vi "WS1050_AD7747_Control_Cap_bank_Measure Ver1.0.vi"(0 "Select Com Port":refnum<visa-resource-name>="COM1", 1 "S_Value C1":dbl, 2 "S_Value C2":dbl, 3 "S_Value C3":dbl, 4 "Push Button to write Offset":bool, 7 "errorin":errorcluster, 8 "Click down to quit":bool, 9 "Push Button to Measue Cap":bool=TRUE, 12 "Mode":bool=TRUE, 14 "Push Button to Initialize AD7747":bool, 15 "CApDac_values":string[](array[string])=["900b99", "900b99", "900b9b"], 16 "Push Button to Calibrate":bool) -> (17 "Com Port Out":refnum<visa-resource-name>="COM1", 20 "C2(pF)":dbl, 21 "C1_Mesa(pF)":dbl, 22 "C2_Mesa(pF)":dbl, 23 "C3_Mesa(pF)":dbl, 24 "C1(pF)":dbl, 25 "C3(pF)":dbl, 27 "error out":errorcluster)   [LabVIEW 2017]
panel:
  # "AD7747 Control Ver1.0"
  # "Interface PIC I2C Control"
  # "Bank Cap Measurements"
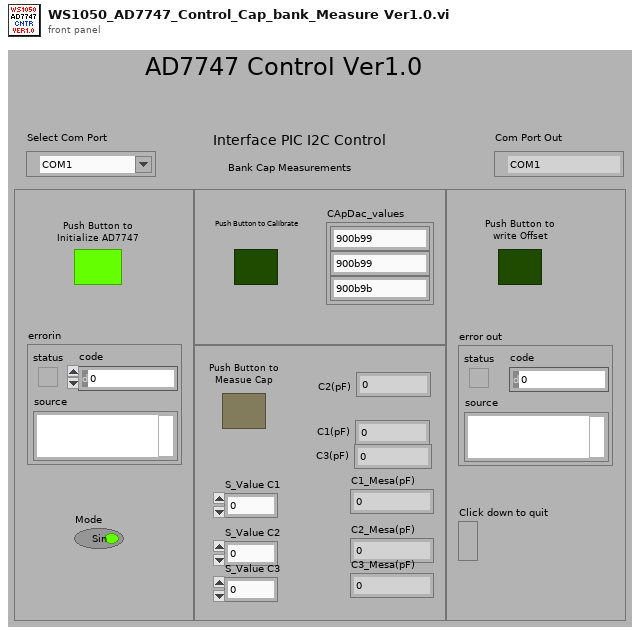
[diagram p1: front panel]
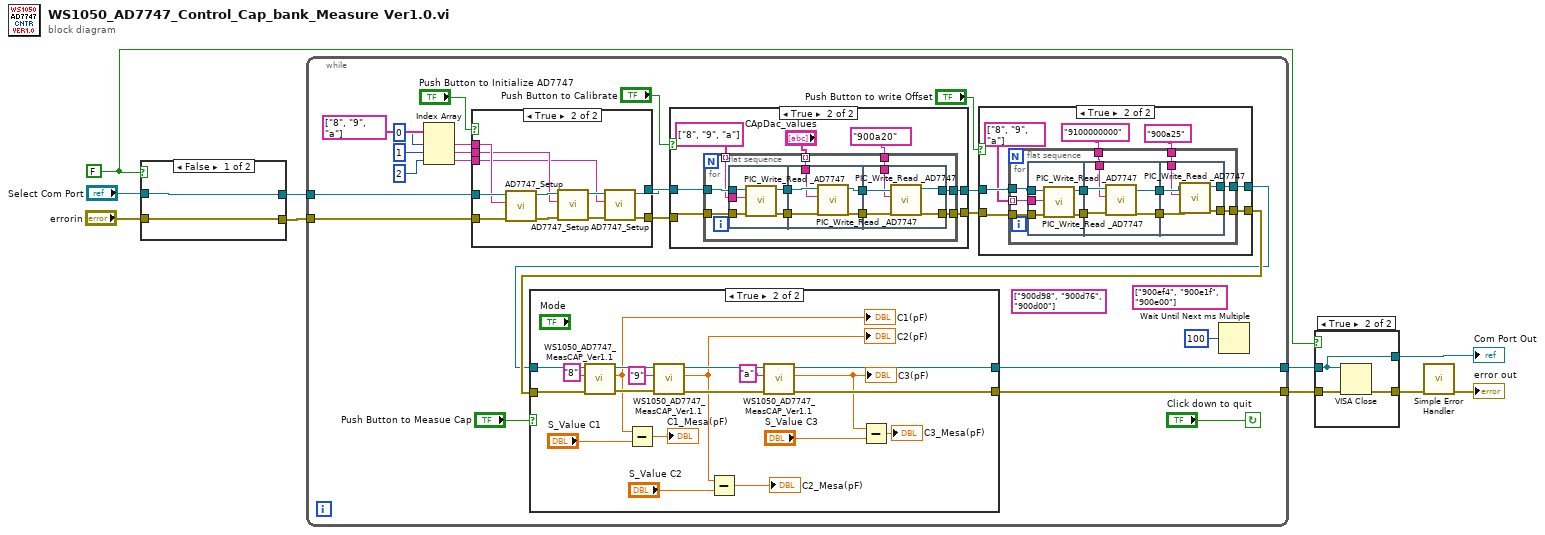
[diagram p0: block diagram]
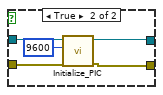
[diagram p3: hidden frame]
diagram:
  w5 = FALSE
  n1 = case shown="False" w5 {
    tunnel: [w11 w17] -> w10
    tunnel: [w12 w16] -> w9
    tunnel: "Select Com Port" -> [w12 w15]
    tunnel: "errorin" -> [w11 w13]
    frame False {
    }
    frame True {
      n2 = call "Initialize_PIC.vi"("error in (no error)"=w13, "baud rate"=u32 9600, "Select Com Port"=w15) -> ("error out"=w17:errorcluster, "VISA resource name out"=w16:refnum<visa-resource-name>)  [unwired: 7 in]
    }
  }
  n3 = while {
    tunnel: w10 -> [w35]
    tunnel: w9 -> [w33]
    tunnel: [w22] -> w8
    tunnel: [w40] -> w7
    stop <- "Click down to quit" continue-if-true
    (unwired) string[] ["900ef4", "900e1f", "900e00"]
    (unwired) string[] ["900d98", "900d76", "900d00"]
    n4 = Index Array(array=string[] ["8", "9", "a"], index #1=0 ("index"), index #2=1 ("index"), index #3=2 ("index")) -> (element #1=w36:string, element #2=w29:string, element #3=w28:string)
    n5 = case shown="True" "Push Button to Initialize AD7747" {
      tunnel: w35 -> [w111 w122]
      tunnel: [w111 w112] -> w23
      tunnel: w33 -> [w110 w121]
      tunnel: w36 -> [_ w116]
      tunnel: w29 -> [_ w115]
      tunnel: w28 -> [_ w114]
      tunnel: [w110 w113] -> w20
      frame False {
      }
      frame True {
        n6 = call "AD7747_Setup.vi"("error in"=w122, "AD7747_Number"=w116, "Control"=w121) -> ("error out"=w120:errorcluster, "Control out"=w119:refnum<visa-resource-name>)  [unwired: 6 in, 1 out]
        n7 = call "AD7747_Setup.vi"("error in"=w120, "AD7747_Number"=w115, "Control"=w119) -> ("error out"=w118:errorcluster, "Control out"=w117:refnum<visa-resource-name>)  [unwired: 6 in, 1 out]
        n8 = call "AD7747_Setup.vi"("error in"=w118, "AD7747_Number"=w114, "Control"=w117) -> ("error out"=w112:errorcluster, "Control out"=w113:refnum<visa-resource-name>)  [unwired: 6 in, 1 out]
      }
    }
    n9 = case shown="True" "Push Button to Calibrate" {
      tunnel: [w76 w84] -> w34
      tunnel: w23 -> [w76 w81]
      tunnel: w20 -> [w77 w80]
      tunnel: [w77 w79] -> w19
      frame False {
      }
      frame True {
        n10 = for {
          tunnel: [w90] -> w84
          tunnel: w80 -> [w94]
          tunnel: w81 -> [w95]
          tunnel: string[] ["8", "9", "a"] -> [w93] mode=indexing
          tunnel: "CApDac_values" -> [w89] mode=indexing
          tunnel: [w88] -> w79
          tunnel: "900a20" ("Data_In 2") -> [w85]
          n11 = flat-sequence {
            tunnel: w95 -> [w100]
            tunnel: w94 -> [w98]
            tunnel: w93 -> [w96]
            tunnel: [w99] -> w92
            tunnel: [w97] -> w91
            tunnel: w92 -> [w104]
            tunnel: w91 -> [w105]
            tunnel: w89 -> [w102]
            tunnel: [w103] -> w87
            tunnel: [w101] -> w86
            tunnel: [w107] -> w88
            tunnel: [w109] -> w90
            tunnel: w87 -> [w109]
            tunnel: w86 -> [w108]
            tunnel: w85 -> [w106]
            frame #0 {
              n12 = call "PIC_Write_Read _AD7747.vi"("error in (no error)"=w100, "command"=w96, "Control"=w98) -> ("error out"=w99:errorcluster, "Control out"=w97:refnum<visa-resource-name>)  [unwired: 6 in, 1 out]
            }
            frame #1 {
              n13 = call "PIC_Write_Read _AD7747.vi"("error in (no error)"=w104, "command"=w102, "Control"=w105) -> ("error out"=w103:errorcluster, "Control out"=w101:refnum<visa-resource-name>)  [unwired: 6 in, 1 out]
            }
            frame #2 {
              n14 = call "PIC_Write_Read _AD7747.vi"("command"=w106, "Control"=w108) -> ("Control out"=w107:refnum<visa-resource-name>)  [unwired: 7 in, 2 out]
            }
          }
        }
      }
    }
    n15 = case shown="True" "Push Button to write Offset" {
      tunnel: w19 -> [w41 w48]
      tunnel: w34 -> [w42 w49]
      tunnel: [w42 w46] -> w21
      tunnel: [w41 w45] -> w18
      frame False {
      }
      frame True {
        n16 = for {
          tunnel: w49 -> [w50]
          tunnel: [w54] -> w46
          tunnel: w48 -> [w60]
          tunnel: string[] ["8", "9", "a"] -> [w59] mode=indexing
          tunnel: "9100000000" ("Data_In 2") -> [w53]
          tunnel: "900a25" ("Data_In 2") -> [w52]
          tunnel: [w51] -> w45
          n17 = flat-sequence {
            tunnel: w60 -> [w63]
            tunnel: w59 -> [w62]
            tunnel: [w65] -> w58
            tunnel: [w64] -> w57
            tunnel: w50 -> [w61]
            tunnel: w58 -> [w68]
            tunnel: w57 -> [w70]
            tunnel: [w67] -> w56
            tunnel: [w69] -> w55
            tunnel: w53 -> [w66]
            tunnel: w56 -> [w74]
            tunnel: w55 -> [w75]
            tunnel: [w73] -> w54
            tunnel: w52 -> [w72]
            tunnel: [w71] -> w51
            frame #0 {
              n18 = call "PIC_Write_Read _AD7747.vi"("error in (no error)"=w61, "command"=w62, "Control"=w63) -> ("error out"=w65:errorcluster, "Control out"=w64:refnum<visa-resource-name>)  [unwired: 6 in, 1 out]
            }
            frame #1 {
              n19 = call "PIC_Write_Read _AD7747.vi"("error in (no error)"=w68, "command"=w66, "Control"=w70) -> ("error out"=w67:errorcluster, "Control out"=w69:refnum<visa-resource-name>)  [unwired: 6 in, 1 out]
            }
            frame #2 {
              n20 = call "PIC_Write_Read _AD7747.vi"("error in (no error)"=w74, "command"=w72, "Control"=w75) -> ("error out"=w73:errorcluster, "Control out"=w71:refnum<visa-resource-name>)  [unwired: 6 in, 1 out]
            }
          }
        }
      }
    }
    n21 = case shown="True" "Push Button to Measue Cap" {
      tunnel: w21 -> [w124 w144]
      tunnel: w18 -> [w123 w143]
      tunnel: [w124 w135] -> w22
      tunnel: [w123 w134] -> w40
      frame False {
      }
      frame True {
        n22 = call "WS1050_AD7747_MeasCAP_Ver1.1.vi"("error in (no error)"=w144, "AD7747_Number"="8", "Control"=w143) -> ("error"=w140:errorcluster, "CAP (pF)"=w132:dbl, "Control out"=w139:refnum<visa-resource-name>)  [unwired: 4 in, 2 out]
        "C1(pF)" <- w132
        n23 = Subtract(x=w132, y="S_Value C1") -> (x-y=→"C1_Mesa(pF)":dbl)
        n24 = call "WS1050_AD7747_MeasCAP_Ver1.1.vi"("error in (no error)"=w140, "AD7747_Number"="9", "Control"=w139) -> ("error"=w137:errorcluster, "CAP (pF)"=w130:dbl, "Control out"=w136:refnum<visa-resource-name>)  [unwired: 4 in, 2 out]
        "C2(pF)" <- w130
        n25 = Subtract(x=w130, y="S_Value C2") -> (x-y=→"C2_Mesa(pF)":dbl)
        n26 = call "WS1050_AD7747_MeasCAP_Ver1.1.vi"("error in (no error)"=w137, "AD7747_Number"="a", "Control"=w136) -> ("error"=w135:errorcluster, "CAP (pF)"=w128:dbl, "Control out"=w134:refnum<visa-resource-name>)  [unwired: 4 in, 2 out]
        "C3(pF)" <- w128
        n27 = Subtract(x=w128, y="S_Value C3") -> (x-y=→"C3_Mesa(pF)":dbl)
      }
    }
    n28 = Wait Until Next ms Multiple(millisecond multiple=u32 100) -> ()  [unwired: 1 out]
  }
  n29 = case shown="True" w5 {
    tunnel: w8 -> [w145 w149]
    tunnel: w7 -> [w146 w148]
    tunnel: [w146 w148] -> w4
    tunnel: [w145 w147] -> w2
    frame False {
    }
    frame True {
      n30 = VISA Close(VISA resource name=w148, error in (no error)=w149) -> (error out=w147:errorcluster)
    }
  }
  "Com Port Out" <- w4
  n31 = call <vilib>:"Simple Error Handler.vi"("error in (no error)"=w2) -> ("error out"=→"error out":errorcluster)  [unwired: 1 in, 7 out]
